vi "Launcher2.0.vi"() -> ()   [LabVIEW 2014]
uses:
  Project/Framework/ActorMeter/ActorMeter.lvclass
  Project/Framework/ActorMeter/ActorMeter.lvclass/ActorMeter.ctl
  <vilib>/ActorFramework/Actor/Actor.lvclass
panel:
  out "Description":string
  in  "Start":bool
  in  "Stop":bool
  in  "Select configuration":u16(ring) items=["Agilent without Stepper", "Agilent", "Simulation 1D", "Simulation 2D", "SolarSystem M266 ISP", "SolarSystem M266", "Videoscan without Stepper", "Videoscan"]
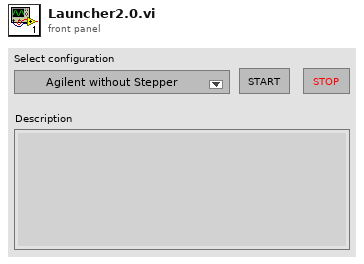
[diagram p1: front panel]
types:
  T1 = typedef "Configuration.ctl" = cluster{"type":string, "name":string}[]
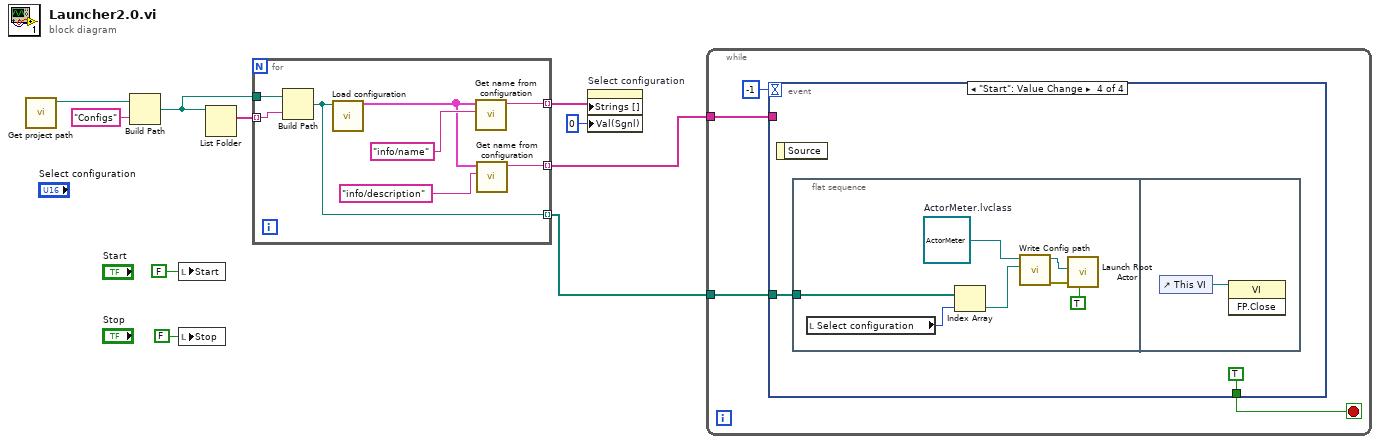
[diagram p0: block diagram]
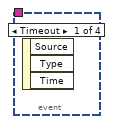
[diagram p2: hidden frame]
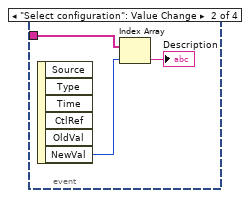
[diagram p3: hidden frame]
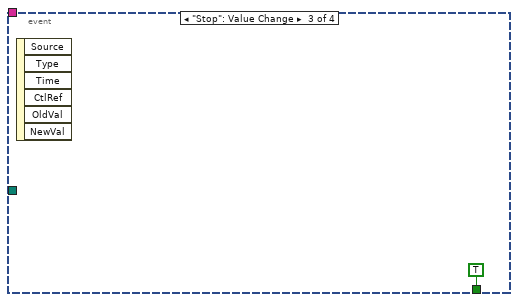
[diagram p4: hidden frame]
diagram:
  n1 = call "Get project path.vi"() -> ("Project path"=w2:path)  [unwired: 11 in]
  n2 = Build Path(base path=w2, name or relative path="Configs") -> (appended path=w9:path)
  n3 = local write "Start"(FALSE ("Start")) -> ()
  n4 = local write "Stop"(FALSE ("Start")) -> ()
  n5 = List Folder(path=w9) -> (filenames=w8:string[])  [unwired: 3 in, 3 out]
  n6 = for {
    tunnel: w9 -> [w18]
    tunnel: w8 -> [w17] mode=indexing
    tunnel: [w13] -> w7 mode=indexing
    tunnel: [w12] -> w6 mode=indexing
    tunnel: [w11] -> w1 mode=indexing
    n7 = Build Path(base path=w18, name or relative path=w17) -> (appended path=w11:path)
    n8 = call "Load configuration.vi"("Path"=w11) -> ("Configuration"=w14:T1)  [unwired: 9 in, 1 out]
    n9 = call "Get name from configuration.vi"("Configuration"=w14, "Type"="info/name") -> ("Name"=w13:string)  [unwired: 7 in, 1 out]
    n10 = call "Get name from configuration.vi"("Configuration"=w14, "Type"="info/description") -> ("Name"=w12:string)  [unwired: 7 in, 1 out]
  }
  n11 = property on="Select configuration" class="Ring (strict)"("Strings []"=w7, "Val(Sgnl)"=u16 0 ("Value (Signaling)")) -> ()  [unwired: 2 in, 2 out]
  n12 = while {
    tunnel: w6 -> [w20]
    tunnel: w1 -> [w19]
    stop <- w21 stop-if-true
    n13 = event shown="[3] \"Start\": Value Change" {
      selector: _ -> [_ _ _ _]
      dyn-events: _ -> [_ _ _ _]
      timeout: -1 -> [_ _ _ _]
      tunnel: [_ _ TRUE TRUE] -> w21
      tunnel: w20 -> [_ w25 _ _]
      tunnel: w19 -> [_ _ _ w27]
      event Timeout {
        n14 = event-data() -> ()  [unwired: 1 in, 3 out]
      }
      event "Select configuration": Value Change {
        n15 = event-data() -> ("NewVal"=w24:u16)  [unwired: 1 in, 5 out]
        n16 = Index Array(array=w25, index=w24) -> (element=→"Description":string)
      }
      event "Stop": Value Change {
        n17 = event-data() -> ()  [unwired: 1 in, 6 out]
      }
      event "Start": Value Change {
        n18 = event-data() -> ()  [unwired: 1 in, 1 out]
        n19 = flat-sequence {
          tunnel: w27 -> [w29]
          frame #0 {
            w33 = refnum<class "ActorMeter.lvclass"> refnum  # ActorMeter.lvclass
            n20 = local read "Select configuration"() -> (w31:u16)
            n21 = Index Array(array=w29, index=w31) -> (element=w30:path)
            n22 = call "Write Config path.vi"("Config path"=w30, "ActorMeter in"=w33) -> ("error out"=w32:errorcluster, "ActorMeter out"=w34:refnum<class "ActorMeter.lvclass">)  [unwired: 8 in]
            n23 = call <vilib>:"Launch Root Actor.vi"("Open Actor Core front panel? (F)"=TRUE, "error in (no error)"=w32, "Actor"=w34) -> ()  [unwired: 7 in, 2 out]
          }
          frame #1 {
            n24 = control-ref of="This VI"() -> (w36:refnum<vi>)
            n25 = invoke class="VI" method="FP.Close"(reference=w36) -> ()  [unwired: 2 in, 3 out]
          }
        }
      }
    }
  }
